vi "Create CSV from TDMS.vi"() -> ()   [LabVIEW 2021, in "PMIC Common.lvlib"]
uses:
  PMIC Common.lvlib
  <vilib>/Utility/file.llb/Write Delimited Spreadsheet (DBL).vi
  <vilib>/Utility/file.llb/Write Delimited Spreadsheet (string).vi
panel:
  in  "Group Names":string[](array[string])=["DCPower Data", "Scope Data"]
  in  "TDMS File Path":path=path "C:/Users/NIJ ASE/Desktop/results/Load Transient Response Vin_12.000 Iout1_2.000 Iout2_3.000.tdms"
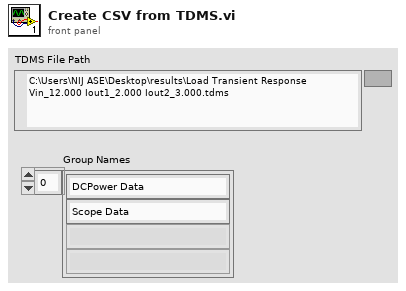
[diagram p1: front panel]
types:
  T1 = enum16{"open", "open or create", "create or replace", "create", "open (read-only)"}
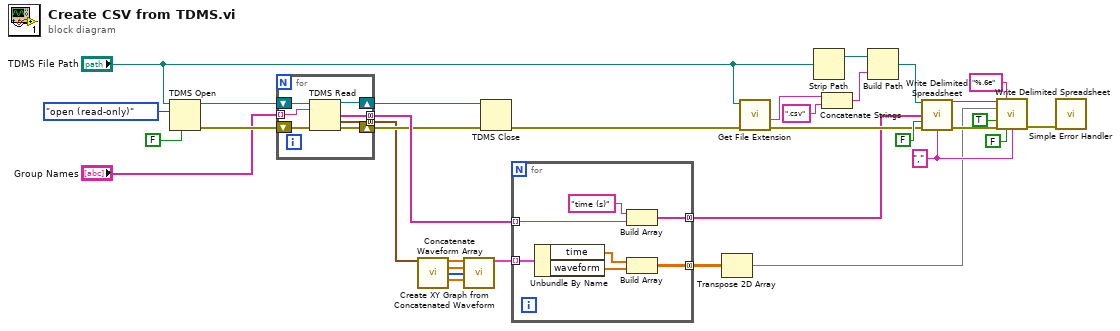
[diagram p0: block diagram]
diagram:
  w28 = "," ("delimiter (\\t)")
  n1 = TDMS Open(6:FALSE ("disable buffering? (T)"), 10:T1."open (read-only)" ("operation (0:open)"), 11:"TDMS File Path") -> (0:w13:errorcluster, 3:w14:refnum<k34>)  [unwired: 4 in]
  n2 = for {
    tunnel: [w38] -> w6 mode=concatenating
    tunnel: [w37] -> w12 mode=concatenating
    shift-right: [w36] -> w11
    shift-left: w14 -> [w40]
    shift-right: [w35] -> w10
    shift-left: w13 -> [w39]
    tunnel: "Group Names" -> [w34] mode=indexing
    n3 = TDMS Read(0:w40, 5:w34, 11:w39) -> (4:w36:refnum<k34>, 8:w37:string[], 10:w38:waveform(dbl)[], 15:w35:errorcluster)  [unwired: 5 in, 2 out]
  }
  n4 = call "Concatenate Waveform Array.vi"("waveform array"=w6) -> ("waveform t0 array"=w5:dbl[], "waveform dt array"=w4:dbl[], "waveform length array"=w3:i32[], "concatenated waveform Y"=w2:dbl[])  [unwired: 11 in]
  n5 = call "Create XY Graph from Concatenated Waveform.vi"("waveform t0 array"=w5, "waveform dt array"=w4, "waveform length array"=w3, "concatenated waveform Y"=w2) -> ("XY Graph Array"=w1:cluster{"time":dbl[], "waveform":dbl[]}[])  [unwired: 11 in]
  n6 = TDMS Close(8:w10, 11:w11) -> (0:w22:errorcluster)  [unwired: 1 out]
  n7 = for {
    tunnel: w12 -> [w44] mode=indexing
    tunnel: w1 -> [w47] mode=indexing
    tunnel: [w42] -> w8 mode=concatenating
    tunnel: [w41] -> w7 mode=concatenating
    n8 = Unbundle By Name(w47) -> ("time"=w46:dbl[], "waveform"=w45:dbl[])
    n9 = Build Array("time (s)" ("element"), w44) -> (w42:string[])
    n10 = Build Array(w46, w45) -> (w41:dbl[][])
  }
  n11 = Transpose 2D Array(2D array=w7) -> (transposed array=w24:dbl[][])
  n12 = call <vilib>:"Get File Extension.vi"("error in (no error)"=w22, "file"="TDMS File Path") -> ("error out"=w21:errorcluster, "filename without extension"=w18:string)  [unwired: 5 in, 3 out]
  n13 = Strip Path(path="TDMS File Path") -> (stripped path=w19:path)  [unwired: 1 out]
  n14 = Concatenate Strings(w18, ".csv" ("string")) -> (w16:string)
  n15 = Build Path(base path=w19, name or relative path=w16) -> (appended path=w15:path)
  n16 = call-poly <vilib>:"Write Delimited Spreadsheet.vi"("file path (dialog if empty)"=w15, "1D data"=w8, "append to file? (new file:F)"=FALSE, "error in (no error)"=w21, "delimiter (\\t)"=w28) -> ("new file path (Not A Path if cancelled)"=w29:path, "error out"=w30:errorcluster)  [unwired: 9 in]
  n17 = call-poly <vilib>:"Write Delimited Spreadsheet.vi"("file path (dialog if empty)"=w29, "format (%.3f)"="%.6e", "2D data"=w24, "append to file? (new file:F)"=TRUE, "error in (no error)"=w30, "transpose? (no:F)"=FALSE, "delimiter (\\t)"=w28) -> ("error out"=w23:errorcluster)  [unwired: 7 in, 1 out]
  n18 = call <vilib>:"Simple Error Handler.vi"("error in (no error)"=w23) -> ()  [unwired: 4 in, 5 out]
